vi "Event Zoom.vi"(4 "RefScale":refnum<vi>, 6 "Control Ref":refnum<k24>, 7 "Event Common Data":T1) -> ()   [LabVIEW 2021]
uses:
  G:/LabVIEW VI/GMap/Data/GMap.NET.WindowsForms.dll
  Data/GMap.NET.WindowsForms.dll
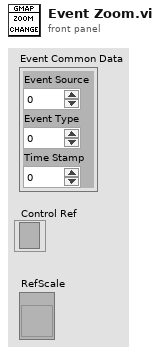
[diagram p1: front panel]
types:
  T1 = cluster{"Event Source":i32, "Event Type":u32, "Time Stamp":u32}
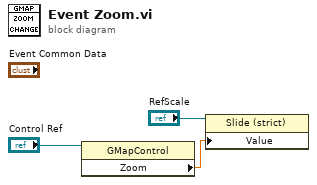
[diagram p0: block diagram]
diagram:
  n1 = property class="GMapControl"(reference="Control Ref") -> ("Zoom"=w1:dbl)  [unwired: 1 in, 2 out]
  n2 = property class="Slide (strict)"(reference="RefScale", "Value"=w1) -> ()  [unwired: 1 in, 2 out]
